vi "Get BufferMap Status.vi"(8 "error in":errorcluster, 11 "BufferMap in":refnum<data-value>) -> (0 "error out":errorcluster, 1 "bufSize":i32, 2 "nbElements":i32, 3 "BufferMap":refnum<data-value>, 4 "full":bool, 5 "Names":string[](array[string]))   [LabVIEW 2013, in "VariantBufferMap.lvclass"]
doc: "This VI returns data from the ring buffer starting from the oldest data and ending with the newest.\n\nThe data is duplicated at the output so this VI allocates new place in the memory for the output."
uses:
  VariantBufferMap.lvclass
  VariantBufferMap.lvclass/VariantBufferMap.ctl
  VariantBuffer/VariantBuffer.lvclass
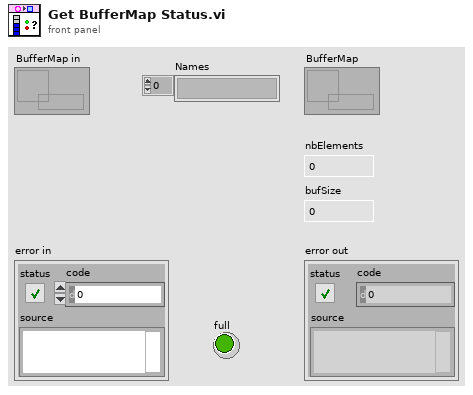
[diagram p1: front panel]
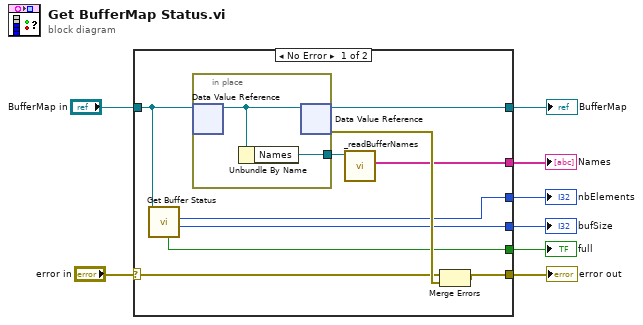
[diagram p0: block diagram]
diagram:
  n1 = case shown="No Error" "error in" {
    selector: "error in" -> [w15 w21]
    tunnel: "BufferMap in" -> [w14 w22]
    tunnel: [w18 w22] -> w7
    tunnel: [w16 w21] -> w4
    tunnel: [w13 _] -> w6
    tunnel: [w11 _] -> w3
    tunnel: [w12 _] -> w2
    tunnel: [w9 _] -> w1
    frame No Error {
      n2 = call "Get Buffer Status.vi"("Buffer in"=w14) -> ("bufSize"=w12:i32, "nbElements"=w13:i32, "full"=w11:bool)  [unwired: 6 in, 2 out]
      n3 = in-place {
        in-place-border: [w19] -> w10
        n4 = in-place-dvr #1(w14) -> (w20:refnum<class "VariantBufferMap.lvclass">)  [unwired: 1 out]
        n5 = Unbundle By Name(w20) -> ("Names"=w19:refnum<data-value>)
        n6 = in-place-dvr #1(w20) -> (w18:refnum<data-value>, w17:errorcluster)
      }
      n7 = call "_readBufferNames.vi"("Data Value Reference in"=w10) -> ("Names"=w9:string[])  [unwired: 9 in, 1 out]
      n8 = Merge Errors(w15, w17) -> (w16:errorcluster)
    }
    frame Error {
    }
  }
  "error out" <- w4
  "BufferMap" <- w7
  "nbElements" <- w6
  "bufSize" <- w2
  "full" <- w3
  "Names" <- w1
